vi "CustomDataTypeScriptingUtilityUI.vi"() -> ()   [LabVIEW 2020]
doc: "Data Type Scripting API Tester."
uses:
  Support/Poly Management/_td_cluster_InstanceInfo.ctl
  Libraries/Data Type Scripting/Data Type Scripting.lvlib
panel:
  out "Module Running?":bool
  in  "Show Block Diagram":bool
  in  "Stop Module":bool
  in  "Start Module":bool
  in  "Hide Module Panel":bool
  in  "Show Module Panel":bool
  in  "Tab Control":T1(tab)
  in  "Poly List":i32(listbox)
  out "Poly Details":T2[](array[typedef])
  in  "Open Poly VI Window":bool
  out "Valid Type":bool
  out "Error Msg":string
  in  "New Selector Name":string caption="Selector Name"
  out "Template Library":path
  in  "Data Type Base Path":path
  in  "New Data Type Name":string caption="Data Type Name"
  in  "New Menu Name":string caption="Menu Name"
  in  "Create New Data Type":bool
  in  "Data Types Edit":i32(listbox)=-1 caption="Data Types"
  in  "Edit Selector Name":string caption="Selector Name"
  in  "Edit Data Type Name":string caption="Data Type Name"
  in  "Edit Menu Name":string caption="Menu Name"
  in  "Update Data Type":bool
  in  "Delete Files":bool=TRUE caption="Delete Data Type Library Files?"
  in  "Data Types":i32(listbox)=-1
  in  "Remove Data Type":bool
  out "Status":string
  # "---FOR DEBUG USE ONLY---"
  # "NOTE: Navigating away from Add New Type and Edit Type will close the type definition and any changes will be lost."
  # "NOTE: \nTo create a hierarchical shortcut menu, use a colon (:) to separate menu items."
  # "NOTE: \nTo create a hierarchical shortcut menu, use a colon (:) to separate menu items."
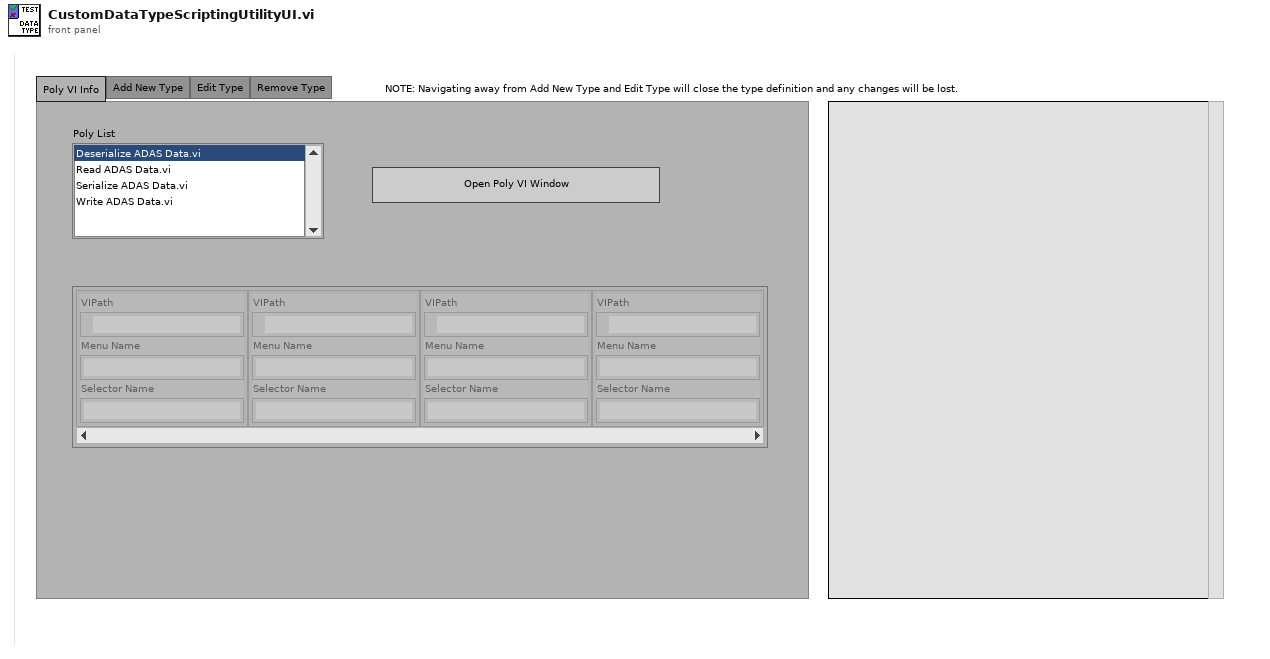
[diagram p1: front panel]
types:
  T1 = enum32{"Poly VI Info", "Add New Type", "Edit Type", "Remove Type"}
  T2 = typedef "_td_cluster_InstanceInfo.ctl" = cluster{"VIPath":path, "Menu Name":string, "Selector Name":string}
  T3 = typedef "Data Type Scripting.lvlib/Broadcast Events--cluster.ctl" = cluster{"Module Did Init":refnum<user-event>, "Status Updated":refnum<user-event>, "Error Reported":refnum<user-event>, "Module Did Stop":refnum<user-event>, "Update Module Execution Status":refnum<user-event>, "Template Path":refnum<user-event>, "Poly List":refnum<user-event>, "Poly Details":refnum<user-event>, "Data Type Valid":refnum<user-event>, "List of Data Types":refnum<user-event>, "Data Type Created":refnum<user-event>, "Selected Edit Data Type Info":refnum<user-event>, "Data Types Base Directory":refnum<user-event>, "Data Type Updated":refnum<user-event>}
  T4 = typedef "LVRectTypeDef.ctl" = cluster{"Left":i16, "Top":i16, "Right":i16, "Bottom":i16}
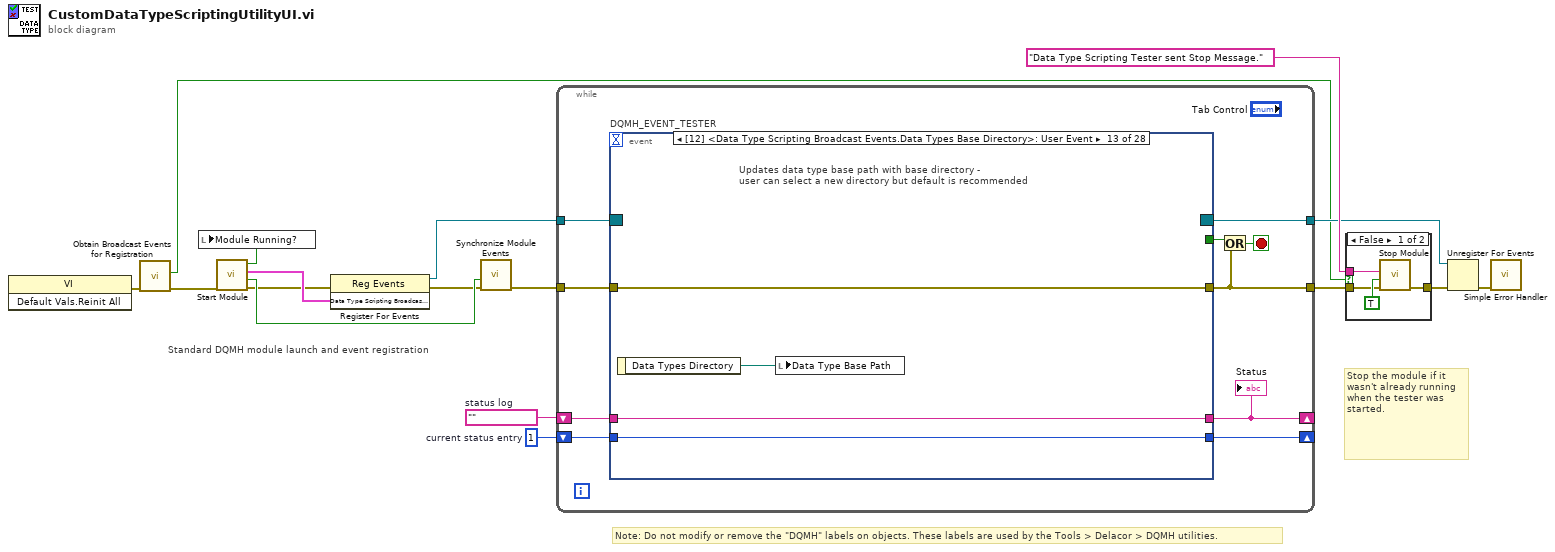
[diagram p0: block diagram]
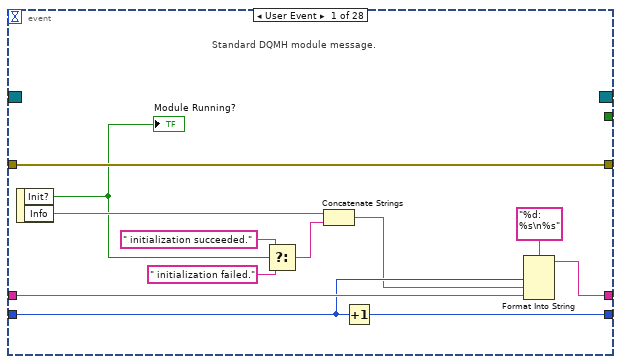
[diagram p3: hidden frame]
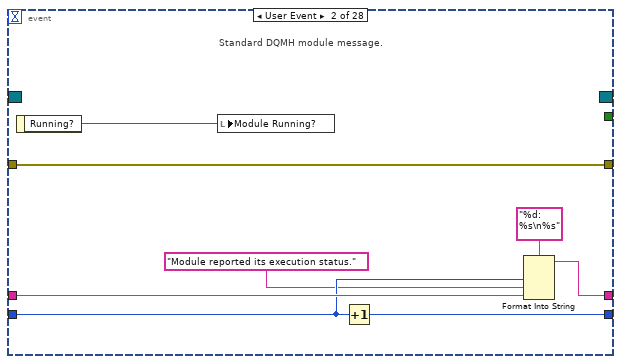
[diagram p4: hidden frame]
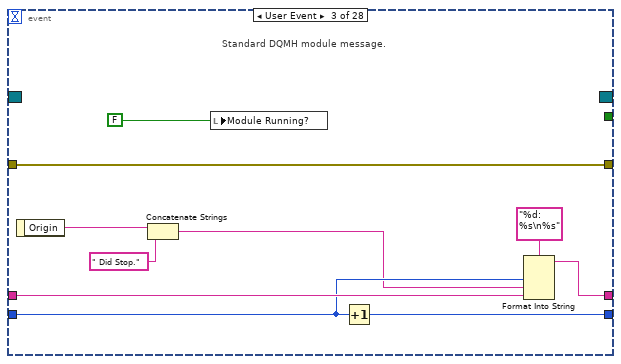
[diagram p5: hidden frame]
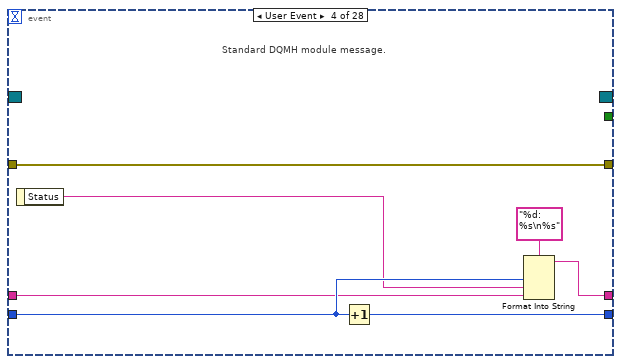
[diagram p6: hidden frame]
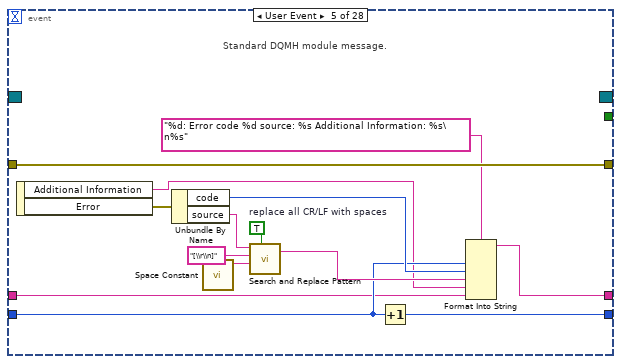
[diagram p7: hidden frame]
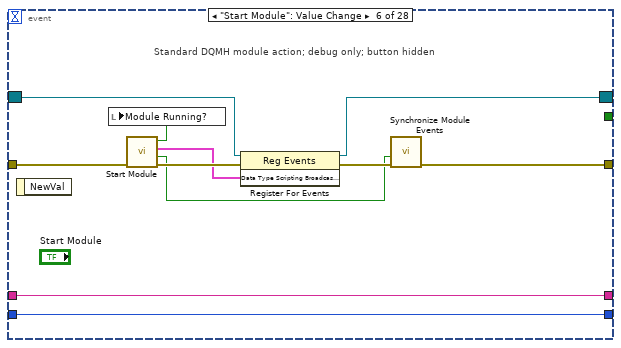
[diagram p8: hidden frame]
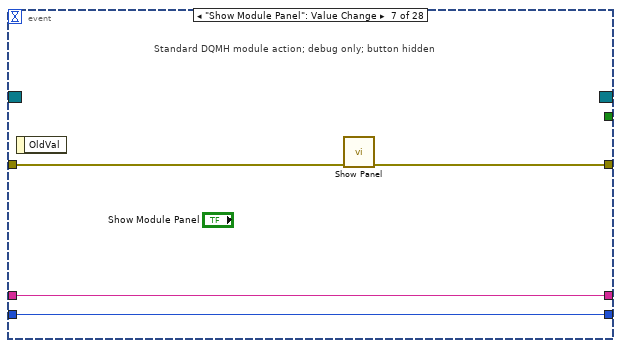
[diagram p9: hidden frame]
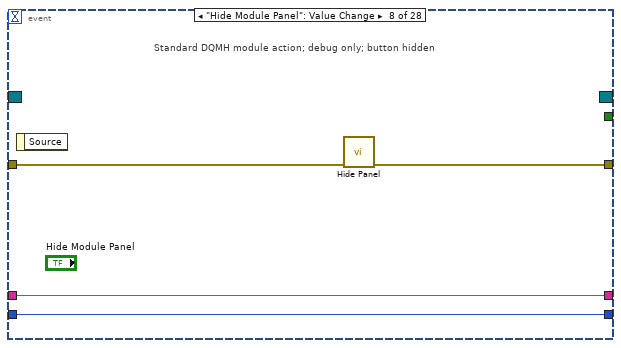
[diagram p10: hidden frame]
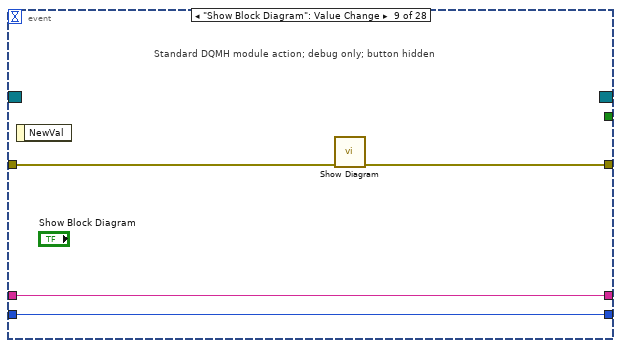
[diagram p11: hidden frame]
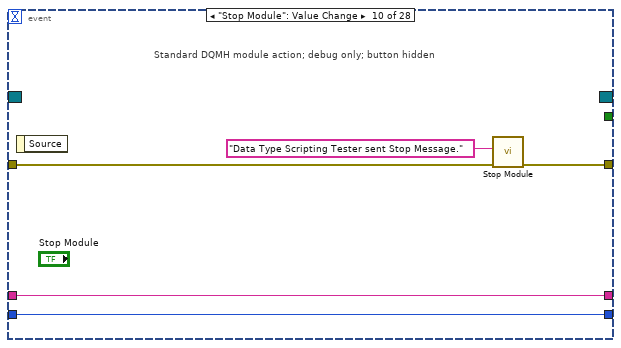
[diagram p12: hidden frame]
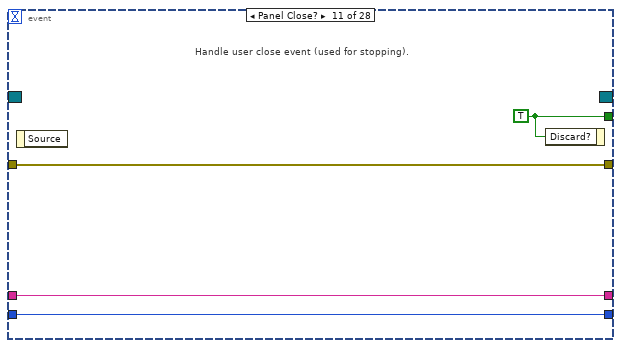
[diagram p13: hidden frame]
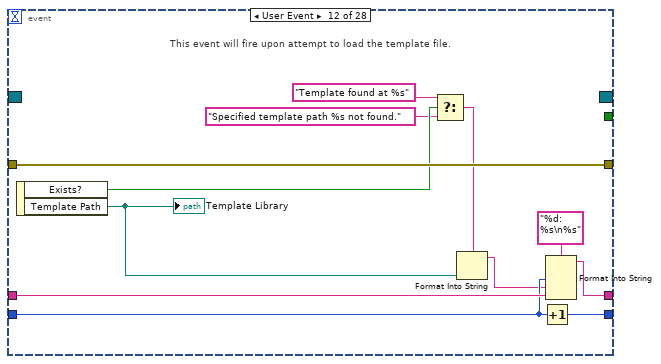
[diagram p14: hidden frame]
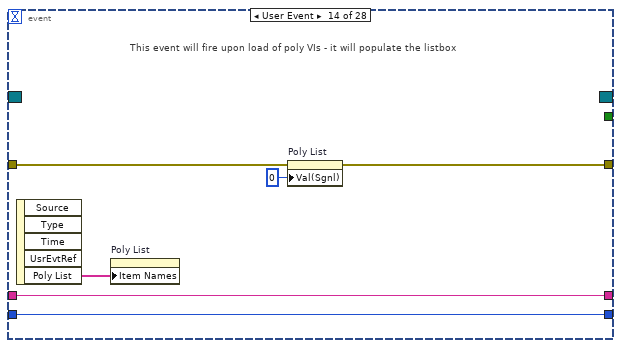
[diagram p15: hidden frame]
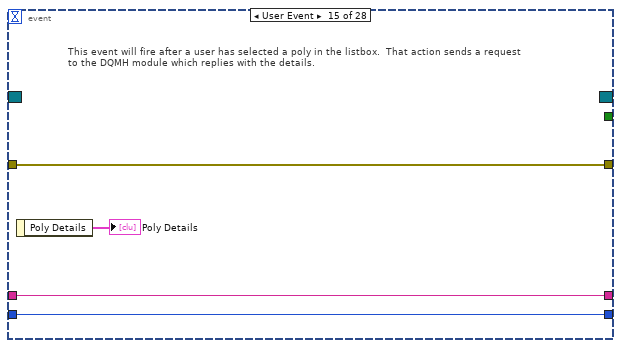
[diagram p16: hidden frame]
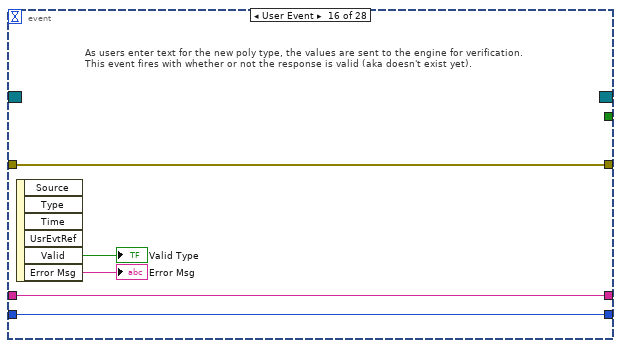
[diagram p17: hidden frame]
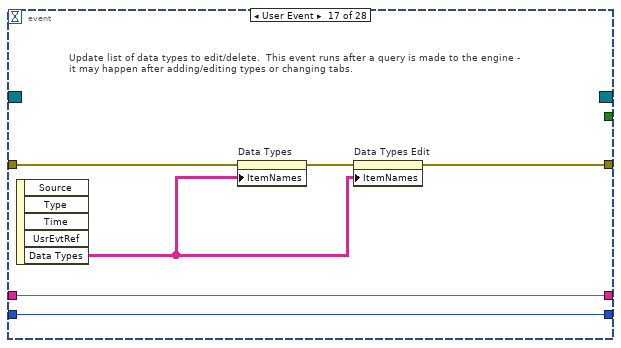
[diagram p18: hidden frame]
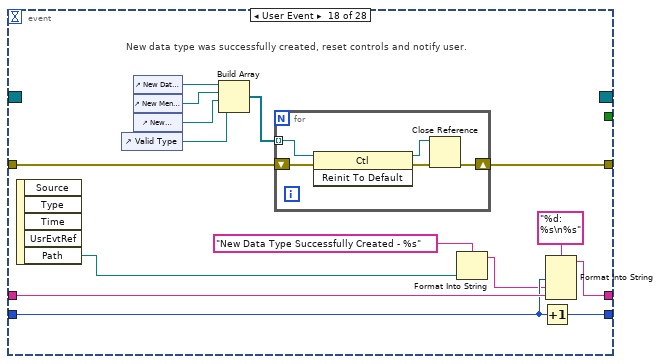
[diagram p19: hidden frame]
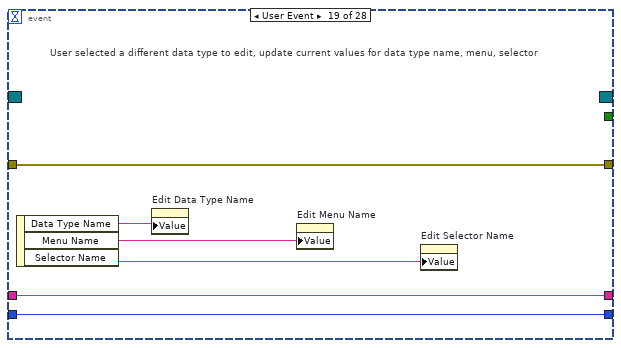
[diagram p20: hidden frame]
diagram:
  w14 = 1  # current status entry
  w15 = ""  # status log
  # "Standard DQMH module launch and event registration"
  # "Stop the module if it wasn't already running when the tester was started."
  # "Note: Do not modify or remove the \"DQMH\" labels on objects. These labels are used by the Tools > Delacor > DQMH utilities."
  n1 = invoke class="VI" method="Default Vals.Reinit All"() -> (error out=w12:errorcluster)  [unwired: 3 in, 2 out]
  n2 = call "Obtain Broadcast Events for Registration.vi"("error in (no error)"=w12) -> ("error out"=w1:errorcluster, "Already running?"=w11:bool)  [unwired: 8 in, 1 out]
  n3 = call "Start Module.vi"("error in (no error)"=w1) -> ("error out"=w5:errorcluster, "Wait for Event Sync?"=w6:bool, "Data Type Scripting Broadcast Events"=w7:T3, "Module Was Already Running?"=w8:bool)  [unwired: 7 in]
  n4 = local write "Module Running?"(w8) -> ()
  n5 = register-events(error in=w5, w7) -> (reference out=w2:refnum<event-registration>, error out=w4:errorcluster)  [unwired: 1 in]
  n6 = call "Synchronize Module Events.vi"("error in"=w4, "Wait for Event Sync?"=w6) -> ("error out"=w3:errorcluster)  [unwired: 9 in]
  n7 = while {
    tunnel: w2 -> [w27]
    tunnel: [w18] -> w10
    shift-right: [w22] -> _
    shift-left: w15 -> [w24]
    shift-right: [w23] -> _
    shift-left: w14 -> [w25]
    tunnel: w3 -> [w20]
    tunnel: [w19] -> w13
    stop <- w21 stop-if-true
    n8 = event "DQMH_EVENT_TESTER" shown="[12] <Data Type Scripting Broadcast Events.Data Types Base Directory>: User Event" {
      selector: w27 -> [_ _ _ _ _ w83 _ _ _ _ _ _ _ _ _ _ _ _ _ _ _ _ _ _ _ _ _ _]
      dyn-events: [_ _ _ _ _ w82 _ _ _ _ _ _ _ _ _ _ _ _ _ _ _ _ _ _ _ _ _ _] -> w19
      timeout: _ -> [_ _ _ _ _ _ _ _ _ _ _ _ _ _ _ _ _ _ _ _ _ _ _ _ _ _ _ _]
      tunnel: [_ _ _ _ _ _ _ _ _ _ w110 _ _ _ _ _ _ _ _ _ _ _ _ _ _ _ _ _] -> w26
      tunnel: [w39 w41 w48 w58 w78 w81 w93 w97 w98 w104 w107 w122 w126 w130 w136 w141 w145 w148 w173 w181 w197 w219 w229 w234 w249 w258 w268 w271] -> w18
      tunnel: w25 -> [w36 w45 w55 w61 w68 w86 w91 w95 w99 w105 w108 w119 w123 w127 w133 w137 w143 w160 w171 w188 w198 w224 w230 w235 w250 w259 w269 w279]
      tunnel: w24 -> [w37 w46 w56 w60 w66 w87 w92 w96 w100 w106 w109 w121 w124 w128 w134 w138 w142 w162 w172 w190 w199 w225 w231 w236 w251 w260 w270 w280]
      tunnel: [w34 w43 w53 w62 w69 w87 w92 w96 w100 w106 w109 w120 w124 w128 w134 w138 w142 w161 w172 w189 w199 w225 w231 w236 w251 w260 w270 w280] -> w22
      tunnel: [w35 w44 w54 w64 w67 w86 w91 w95 w99 w105 w108 w118 w123 w127 w133 w137 w143 w159 w171 w187 w198 w224 w230 w235 w250 w259 w269 w279] -> w23
      tunnel: w20 -> [w39 w41 w48 w58 w78 w80 w90 w94 w101 w102 w107 w122 w126 w131 w136 w141 w147 w149 w173 w176 w200 w221 w232 w237 w252 w261 w263 w278]
      event User Event {
        # "Standard DQMH module message."
        n9 = event-data() -> ("Init?"=w31:bool, "Info"=w33:string)  [unwired: 1 in]
        "Module Running?" <- w31
        n10 = Select(t=" initialization succeeded.", s=w31, f=" initialization failed.") -> (s? t:f=w28:string)
        n11 = Concatenate Strings(w33, w28) -> (w32:string)
        n12 = Increment(x=w36) -> (x+1=w35:i32)
        n13 = Format Into String(format string="%d: %s\n%s", w36, w32, w37) -> (resulting string=w34:string)  [unwired: 2 in, 1 out]
      }
      event User Event {
        # "Standard DQMH module message."
        n14 = event-data() -> ("Running?"=w40:bool)  [unwired: 1 in]
        n15 = local write "Module Running?"(w40) -> ()
        n16 = Increment(x=w45) -> (x+1=w44:i32)
        n17 = Format Into String(format string="%d: %s\n%s", w45, "Module reported its execution status.", w46) -> (resulting string=w43:string)  [unwired: 2 in, 1 out]
      }
      event User Event {
        # "Standard DQMH module message."
        n18 = event-data() -> ("Origin"=w52:string)  [unwired: 1 in]
        n19 = Concatenate Strings(w52, " Did Stop.") -> (w51:string)
        n20 = local write "Module Running?"(FALSE ("Module Did Init?")) -> ()
        n21 = Increment(x=w55) -> (x+1=w54:i32)
        n22 = Format Into String(format string="%d: %s\n%s", w55, w51, w56) -> (resulting string=w53:string)  [unwired: 2 in, 1 out]
      }
      event User Event {
        # "Standard DQMH module message."
        n23 = event-data() -> ("Status"=w59:string)  [unwired: 1 in]
        n24 = Increment(x=w61) -> (x+1=w64:i32)
        n25 = Format Into String(format string="%d: %s\n%s", w61, w59, w60) -> (resulting string=w62:string)  [unwired: 2 in, 1 out]
      }
      event User Event {
        w74 = TRUE  # replace all CR/LF with spaces
        # "Standard DQMH module message."
        n26 = event-data() -> ("Additional Information"=w65:string, "Error"=w70:errorcluster)  [unwired: 1 in]
        n27 = Unbundle By Name(w70) -> ("code"=w71:i32, "source"=w72:string)
        n28 = call <vilib>:"Space Constant.vi"() -> ("String"=w75:string)
        n29 = call <vilib>:"Search and Replace Pattern.vi"("string"=w72, "regular expression (\"\")"="[\\r\\n]" ("regular expression (\"\")"), "replace string (\"\")"=w75, "replace all? (F)"=w74) -> ("result string"=w73:string)  [unwired: 1 in, 1 out]
        n30 = Increment(x=w68) -> (x+1=w67:i32)
        n31 = Format Into String(format string="%d: Error code %d source: %s Additional Information: %s\n%s", w68, w71, w73, w65, w66) -> (resulting string=w69:string)  [unwired: 2 in, 1 out]
      }
      event "Start Module": Value Change {
        # "Standard DQMH module action; debug only; button hidden"
        n32 = event-data() -> ()  [unwired: 1 in, 1 out]
        n33 = call "Start Module.vi"("error in (no error)"=w80) -> ("error out"=w88:errorcluster, "Wait for Event Sync?"=w85:bool, "Data Type Scripting Broadcast Events"=w84:T3, "Module Was Already Running?"=w79:bool)  [unwired: 7 in]
        n34 = local write "Module Running?"(w79) -> ()
        n35 = register-events(reference=w83, error in=w88, w84) -> (reference out=w82:refnum<event-registration>, error out=w89:errorcluster)
        n36 = call "Synchronize Module Events.vi"("error in"=w89, "Wait for Event Sync?"=w85) -> ("error out"=w81:errorcluster)  [unwired: 9 in]
      }
      event "Show Module Panel": Value Change {
        # "Standard DQMH module action; debug only; button hidden"
        n37 = event-data() -> ()  [unwired: 1 in, 1 out]
        n38 = call "Show Panel.vi"("error in (no error)"=w90) -> ("error out"=w93:errorcluster)  [unwired: 10 in]
      }
      event "Hide Module Panel": Value Change {
        # "Standard DQMH module action; debug only; button hidden"
        n39 = event-data() -> ()  [unwired: 1 in, 1 out]
        n40 = call "Hide Panel.vi"("error in (no error)"=w94) -> ("error out"=w97:errorcluster)  [unwired: 10 in]
      }
      event "Show Block Diagram": Value Change {
        # "Standard DQMH module action; debug only; button hidden"
        n41 = event-data() -> ()  [unwired: 1 in, 1 out]
        n42 = call "Show Diagram.vi"("error in (no error)"=w101) -> ("error out"=w98:errorcluster)  [unwired: 10 in]
      }
      event "Stop Module": Value Change {
        # "Standard DQMH module action; debug only; button hidden"
        n43 = event-data() -> ()  [unwired: 1 in, 1 out]
        n44 = call "Stop Module.vi"("error in"=w102, "Origin"="Data Type Scripting Tester sent Stop Message.") -> ("error out"=w104:errorcluster)  [unwired: 9 in]
      }
      event Panel Close? {
        w110 = TRUE ("Discard?")
        # "Handle user close event (used for stopping)."
        n45 = event-data() -> ()  [unwired: 1 in, 1 out]
        n46 = event-data("Discard?"=w110) -> ()  [unwired: 1 in, 1 out]
      }
      event User Event {
        # "This event will fire upon attempt to load the template file."
        n47 = event-data() -> ("Exists?"=w115:bool, "Template Path"=w111:path)  [unwired: 1 in]
        "Template Library" <- w111
        n48 = Select(t="Template found at %s" ("format string"), s=w115, f="Specified template path %s not found." ("format string")) -> (s? t:f=w112:string)
        n49 = Format Into String(format string=w112, w111) -> (resulting string=w116:string)  [unwired: 2 in, 1 out]
        n50 = Increment(x=w119) -> (x+1=w118:i32)
        n51 = Format Into String(format string="%d: %s\n%s", w119, w116, w121) -> (resulting string=w120:string)  [unwired: 2 in, 1 out]
      }
      event User Event {
        # "Updates data type base path with base directory - \nuser can select a new directory but default is recommended"
        n52 = event-data() -> ("Data Types Directory"=w125:path)  [unwired: 1 in]
        n53 = local write "Data Type Base Path"(w125) -> ()
      }
      event User Event {
        # "This event will fire upon load of poly VIs - it will populate the listbox"
        n54 = event-data() -> ("Poly List"=w132:string[])  [unwired: 1 in, 4 out]
        n55 = property on="Poly List" class="LstBox (strict)"("Item Names"=w132) -> ()  [unwired: 2 in, 2 out]
        n56 = property on="Poly List" class="LstBox (strict)"(error in=w131, "Val(Sgnl)"=0 ("Value (Signaling)")) -> (error out=w130:errorcluster)  [unwired: 1 in, 1 out]
      }
      event User Event {
        # "This event will fire after a user has selected a poly in the listbox.  That action sends a request\nto the DQMH module which replies with the details."
        n57 = event-data() -> ("Poly Details"=→"Poly Details":T2[])  [unwired: 1 in]
      }
      event User Event {
        # "As users enter text for the new poly type, the values are sent to the engine for verification.\nThis event fires with whether or not the response is valid (aka doesn't exist yet)."
        n58 = event-data() -> ("Valid"=→"Valid Type":bool, "Error Msg"=→"Error Msg":string)  [unwired: 1 in, 4 out]
      }
      event User Event {
        # "Update list of data types to edit/delete.  This event runs after a query is made to the engine -\nit may happen after adding/editing types or changing tabs."
        n59 = event-data() -> ("Data Types"=w144:string[][])  [unwired: 1 in, 4 out]
        n60 = property on="Data Types" class="MCListbox (strict)"(error in=w147, "ItemNames"=w144) -> (error out=w146:errorcluster)  [unwired: 1 in, 1 out]
        n61 = property on="Data Types Edit" class="MCListbox (strict)"(error in=w146, "ItemNames"=w144) -> (error out=w145:errorcluster)  [unwired: 1 in, 1 out]
      }
      event User Event {
        # "New data type was successfully created, reset controls and notify user."
        n62 = event-data() -> ("Path"=w155:path)  [unwired: 1 in, 4 out]
        n63 = control-ref of="Valid Type"() -> (w150:refnum<vi>)
        n64 = control-ref of="New Data Type Name"() -> (w154:refnum<vi>)
        n65 = control-ref of="New Menu Name"() -> (w153:refnum<vi>)
        n66 = control-ref of="New Selector Name"() -> (w152:refnum<vi>)
        n67 = Build Array(w154, w153, w152, w150) -> (w151:refnum<vi>[])
        n68 = for {
          tunnel: w151 -> [w167] mode=indexing
          shift-right: [w164] -> w148
          shift-left: w149 -> [w163]
          n69 = invoke class="Ctl" method="Reinit To Default"(reference=w167, error in=w163) -> (reference out=w166:refnum<vi>, error out=w165:errorcluster)  [unwired: 1 in, 1 out]
          n70 = Close Reference(reference=w166, error in (no error)=w165) -> (error out=w164:errorcluster)
        }
        n71 = Format Into String(format string="New Data Type Successfully Created - %s", w155) -> (resulting string=w156:string)  [unwired: 2 in, 1 out]
        n72 = Increment(x=w160) -> (x+1=w159:i32)
        n73 = Format Into String(format string="%d: %s\n%s", w160, w156, w162) -> (resulting string=w161:string)  [unwired: 2 in, 1 out]
      }
      event User Event {
        # "User selected a different data type to edit, update current values for data type name, menu, selector"
        n74 = event-data() -> ("Data Type Name"=w170:string, "Menu Name"=w169:string, "Selector Name"=w168:string)  [unwired: 1 in]
        n75 = property on="Edit Data Type Name" class="Str"("Value"=w170) -> ()  [unwired: 2 in, 2 out]
        n76 = property on="Edit Menu Name" class="Str"("Value"=w169) -> ()  [unwired: 2 in, 2 out]
        n77 = property on="Edit Selector Name" class="Str"("Value"=w168) -> ()  [unwired: 2 in, 2 out]
      }
      event User Event {
        # "Data type successfully edited, reset controls and notify user."
        n78 = event-data() -> ("Data Type Library Path"=w180:path)  [unwired: 1 in, 4 out]
        n79 = control-ref of="Edit Data Type Name"() -> (w179:refnum<vi>)
        n80 = control-ref of="Edit Menu Name"() -> (w178:refnum<vi>)
        n81 = control-ref of="Edit Selector Name"() -> (w177:refnum<vi>)
        n82 = Build Array(w179, w178, w177) -> (w174:refnum<vi>[])
        n83 = for {
          shift-right: [w193] -> w175
          shift-left: w176 -> [w195]
          tunnel: w174 -> [w194] mode=indexing
          n84 = invoke class="Str" method="Reinit To Default"(reference=w194, error in=w195) -> (reference out=w191:refnum<vi>, error out=w192:errorcluster)  [unwired: 1 in, 1 out]
          n85 = Close Reference(reference=w191, error in (no error)=w192) -> (error out=w193:errorcluster)
        }
        n86 = call "Get List of Data Types.vi"("error in"=w175) -> ("error out"=w182:errorcluster)  [unwired: 10 in]
        n87 = Format Into String(format string="Data Type Updated - %s", w180) -> (resulting string=w184:string)  [unwired: 2 in, 1 out]
        n88 = property on="Data Types Edit" class="MCListbox (strict)"(error in=w182, "Value"=-1 ("Data Types Edit")) -> (error out=w181:errorcluster)  [unwired: 1 in, 1 out]
        n89 = Increment(x=w188) -> (x+1=w187:i32)
        n90 = Format Into String(format string="%d: %s\n%s", w188, w184, w190) -> (resulting string=w189:string)  [unwired: 2 in, 1 out]
      }
      event "Tab Control": Value Change {
        # "User selected different tab control - take different actions"
        n91 = event-data() -> ("NewVal"=w196:T1)  [unwired: 1 in]
        n92 = case shown="\"Poly VI Info\"" w196 {
          tunnel: w200 -> [w201 w203 w206 w213 w216]
          tunnel: [w201 w204 w209 w210 w217] -> w197
          frame Default {
            # "No actions"
          }
          frame "Poly VI Info" {
            # "Close any open type def; get updated poly list"
            n93 = call "Close Process Data Type Def.vi"("error in"=w203) -> ("error out"=w202:errorcluster)  [unwired: 10 in]
            n94 = call "Get Poly List.vi"("error in"=w202) -> ("error out"=w204:errorcluster)  [unwired: 10 in]
          }
          frame "Add New Type" {
            # "Close any open type def; \nOpen template type def"
            n95 = call "Close Process Data Type Def.vi"("error in"=w206) -> ("error out"=w205:errorcluster)  [unwired: 10 in]
            n96 = property class="VI"(error in=w205) -> (error out=w208:errorcluster, "Front Panel.PanelBounds"=w207:T4)  [unwired: 1 in, 1 out]
            n97 = call "Open Process Data TypeDef.vi"("error in"=w208, "Panel Bounds"=w207) -> ("error out"=w209:errorcluster)  [unwired: 9 in]
          }
          frame "Edit Type" {
            # "Close any open type def;\nUpdate list of types"
            n98 = call "Close Process Data Type Def.vi"("error in"=w213) -> ("error out"=w212:errorcluster)  [unwired: 10 in]
            n99 = call "Get List of Data Types.vi"("error in"=w212) -> ("error out"=w211:errorcluster)  [unwired: 10 in]
            n100 = property on="Data Types Edit" class="MCListbox (strict)"(error in=w211, "Value"=-1 ("Data Types Edit")) -> (error out=w210:errorcluster)  [unwired: 1 in, 1 out]
          }
          frame "Remove Type" {
            # "Close any open type def;\nUpdate list of types"
            n101 = call "Close Process Data Type Def.vi"("error in"=w216) -> ("error out"=w215:errorcluster)  [unwired: 10 in]
            n102 = call "Get List of Data Types.vi"("error in"=w215) -> ("error out"=w217:errorcluster)  [unwired: 10 in]
          }
        }
      }
      event "Poly List": Value Change {
        # "User selected a different poly in the list, send request to get updated details"
        n103 = event-data() -> ("NewVal"=w222:i32)  [unwired: 1 in]
        n104 = property on="Poly List" class="LstBox (strict)"(error in=w221) -> (error out=w220:errorcluster, "Item Names"=w223:string[])  [unwired: 1 in, 1 out]
        n105 = Index Array(array=w223, index=w222) -> (element=w218:string)
        n106 = call "Get Poly Details.vi"("error in"=w220, "Poly VI Name"=w218) -> ("error out"=w219:errorcluster)  [unwired: 9 in]
      }
      event "Open Poly VI Window": Value Change {
        # "User requested a poly VI window be opened; send request to engine"
        n107 = event-data() -> ()  [unwired: 1 in, 1 out]
        n108 = property on="Poly List" class="LstBox (strict)"() -> ("Item Names"=w228:string[])  [unwired: 2 in, 2 out]
        n109 = Index Array(array=w228, index="Poly List") -> (element=w226:string)
        n110 = call "Open Poly VI Window.vi"("error in"=w232, "Poly VI Name"=w226) -> ("error out"=w229:errorcluster)  [unwired: 9 in]
      }
      event "Create New Data Type": Value Change {
        # "If data type is valid (menu/selector/type name is unique), send request to create new type;\notherwise warn user that type is not valid"
        n111 = event-data() -> ()  [unwired: 1 in, 1 out]
        n112 = local read "Valid Type"() -> (w233:bool)
        n113 = case shown="True" w233 {
          tunnel: w237 -> [w239 w245]
          tunnel: [w239 w244] -> w234
          frame False {
            n114 = One Button Dialog(message="Data Type Not Valid.") -> ()  [unwired: 1 in, 1 out]
          }
          frame True {
            n115 = call "Create New Data Type.vi"("Selector"="New Selector Name", "Menu"="New Menu Name", "error in"=w245, "Type Name"="New Data Type Name", "Type Directory"="Data Type Base Path") -> ("error out"=w244:errorcluster)  [unwired: 6 in]
          }
        }
      }
      event "Data Type Base Path", "New Data Type Name", "New Menu Name", "New Selector Name": Value Change {
        # "User has edited menu/selector/data type name/path - send request to verify if unique"
        n116 = event-data() -> ()  [unwired: 1 in, 6 out]
        n117 = local read "New Data Type Name"() -> (w253:string)
        n118 = local read "Data Type Base Path"() -> (w246:path)
        n119 = local read "New Selector Name"() -> (w248:string)
        n120 = local read "New Menu Name"() -> (w247:string)
        n121 = call "Verify New Data Type.vi"("Selector"=w248, "Menu"=w247, "error in"=w252, "Type Name"=w253, "Type Directory"=w246) -> ("error out"=w249:errorcluster)  [unwired: 6 in]
      }
      event "Remove Data Type": Value Change {
        # "User selected remove type, send request to remove"
        n122 = event-data() -> ()  [unwired: 1 in, 1 out]
        n123 = property on="Data Types" class="MCListbox (strict)"() -> ("ItemNames"=w257:string[][])  [unwired: 2 in, 2 out]
        n124 = Index Array(array=w257, index (row)="Data Types") -> (element=w255:string[])  [unwired: 1 in]
        n125 = call "Remove Data Type.vi"("error in"=w261, "Delete Files?"="Delete Files", "Data Type to Remove"=w255) -> ("error out"=w258:errorcluster)  [unwired: 8 in]
      }
      event "Data Types Edit": Value Change {
        # "User selected a different type in the list, send request to get selected type def \nand menu/selector/name values"
        n126 = event-data() -> ()  [unwired: 1 in, 6 out]
        n127 = property class="VI"(error in=w263) -> (error out=w262:errorcluster, "Front Panel.PanelBounds"=w264:T4)  [unwired: 1 in, 1 out]
        n128 = property on="Data Types Edit" class="MCListbox (strict)"() -> ("ItemNames"=w266:string[][])  [unwired: 2 in, 2 out]
        n129 = Index Array(array=w266, index (row)="Data Types Edit") -> (element=w265:string[])  [unwired: 1 in]
        n130 = call "Load Edit Data Type.vi"("error in"=w262, "Data Type"=w265, "Panel Bounds"=w264) -> ("error out"=w268:errorcluster)  [unwired: 8 in]
      }
      event "Update Data Type": Value Change {
        # "User selected edit type; send request to update type"
        n131 = event-data() -> ()  [unwired: 1 in, 6 out]
        n132 = local read "Data Types Edit"() -> (w273:i32)
        n133 = property on="Data Types Edit" class="MCListbox (strict)"() -> ("ItemNames"=w274:string[][])  [unwired: 2 in, 2 out]
        n134 = Index Array(array=w274, index (row)=w273) -> (element=w272:string[])  [unwired: 1 in]
        n135 = call "Edit Update Data Type.vi"("Selected Data Type"=w272, "New Selector Name"="Edit Selector Name", "error in"=w278, "New Menu Name"="Edit Menu Name", "New Data Type Name"="Edit Data Type Name") -> ("error out"=w271:errorcluster)  [unwired: 6 in]
      }
    }
    "Status" <- w22
    n136 = Or(x=w26, y=w18) -> (x .or. y?=w21:bool)
  }
  n137 = case shown="False" w11 {
    tunnel: [w284 w285] -> w17
    tunnel: "Data Type Scripting Tester sent Stop Message." ("Origin") -> [w283 _]
    tunnel: w10 -> [w281 w285]
    frame False {
      n138 = call "Stop Module.vi"("error in"=w281, "Wait for Module to Stop? (F)"=TRUE ("Wait for Module to stop?"), "Origin"=w283) -> ("error out"=w284:errorcluster)  [unwired: 8 in]
    }
    frame True {
    }
  }
  n139 = Unregister For Events(event registration refnum=w13, error in=w17) -> (error out=w9:errorcluster)
  n140 = call <vilib>:"Simple Error Handler.vi"("error in (no error)"=w9) -> ()  [unwired: 4 in, 5 out]
